vi "CtlRefToJson.vi"(8 "error (in)":errorcluster, 10 "Destination Directory":path, 11 "vi reference":refnum<vi>) -> (0 "error out":errorcluster, 1 "JSON File Path":path, 3 "String":string)   [LabVIEW 2017]
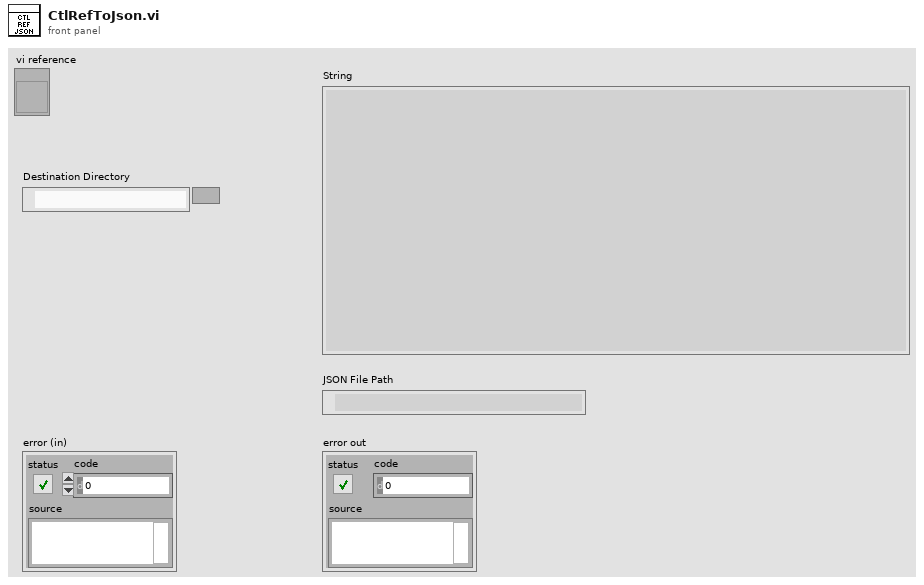
[diagram p1: front panel]
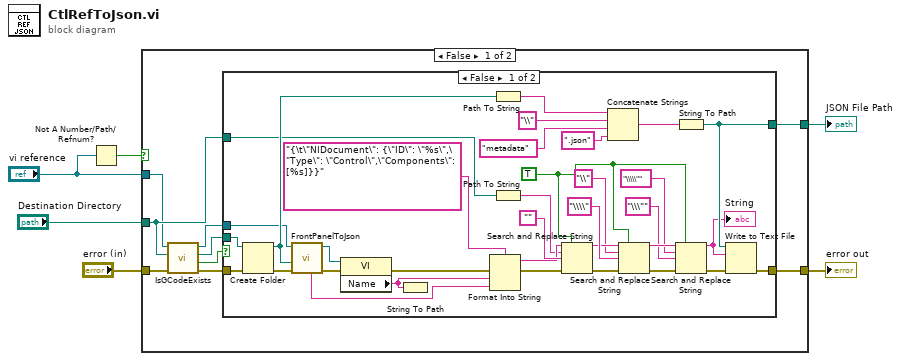
[diagram p0: block diagram]
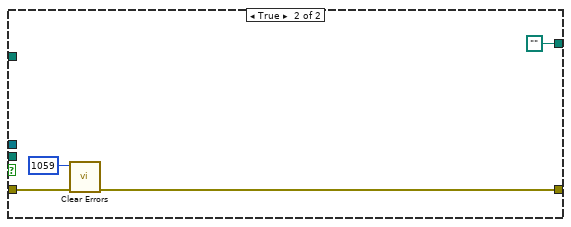
[diagram p2: hidden frame]
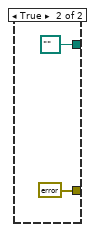
[diagram p3: hidden frame]
diagram:
  n1 = Not A Number/Path/Refnum?(number/path/refnum="vi reference") -> (NaN/Path/Refnum?=w2:bool)
  n2 = case shown="False" w2 {
    tunnel: [w15 path ""] -> w6
    tunnel: [w14 errorcluster {"status"=FALSE, "code"=0, "source"=""} ("error out")] -> w5
    tunnel: "error (in)" -> [w13 _]
    tunnel: "Destination Directory" -> [w10 _]
    tunnel: "vi reference" -> [w9 _]
    frame False {
      n3 = call "IsGCodeExists.vi"("error in (no error)"=w13, "Destination Directory"=w10, "VI (in)"=w9) -> ("error out"=w11:errorcluster, "file or folder exists?"=w12:bool, "VI Folder"=w7:path, "VI (out)"=w8:refnum<vi>)  [unwired: 3 in]
      n4 = case shown="False" w12 {
        tunnel: [w49 path ""] -> w15
        tunnel: [w27 w53] -> w14
        tunnel: w10 -> [w20 _]
        tunnel: w8 -> [w30 _]
        tunnel: w11 -> [w29 w50]
        tunnel: w7 -> [w28 _]
        frame False {
          w21 = TRUE ("replace all? (F)")
          n5 = Create Folder(path (use dialog)=w28, error in=w29) -> (created path=w34:path, error out=w32:errorcluster)  [unwired: 1 in, 1 out]
          n6 = call "FrontPanelToJson.vi"("error in"=w32, "VI Path"=w34, "VI in"=w30) -> ("error out"=w31:errorcluster, "VI out"=w18:refnum<vi>, "JSON"=w33:string)  [unwired: 5 in]
          n7 = property class="VI"(reference=w18, error in=w31) -> (error out=w40:errorcluster, "Name"=w17:string)  [unwired: 1 out]
          n8 = String To Path(string=w17) -> ()  [unwired: 1 out]
          n9 = Format Into String(format string="{\t\"NIDocument\": {\"ID\": \"%s\",\"Type\": \"Control\",\"Components\": [%s]}}", error in=w40, w17, w33) -> (resulting string=w44:string, error out=w38:errorcluster)  [unwired: 1 in]
          n10 = Path To String(path=w34) -> (string=w39:string)
          n11 = Path To String(path=w20) -> (string=w35:string)
          n12 = Search and Replace String(replace all?=w21, input string=w44, search string=w35, replace string="", error in=w38) -> (result string=w45:string, error out=w37:errorcluster)  [unwired: 3 in, 2 out]
          n13 = Concatenate Strings(w39, "\\" ("string"), "metadata" ("string"), ".json" ("string")) -> (w48:string)
          n14 = Search and Replace String(replace all?=w21, input string=w45, search string="\\", replace string="\\\\" ("replace string (\"\")"), error in=w37) -> (result string=w26:string, error out=w22:errorcluster)  [unwired: 3 in, 2 out]
          n15 = String To Path(string=w48) -> (path=w49:path)
          n16 = Search and Replace String(replace all?=w21, input string=w26, search string="\\\\\"", replace string="\\\"" ("replace string (\"\")"), error in=w22) -> (result string=w25:string, error out=w19:errorcluster)  [unwired: 3 in, 2 out]
          "String" <- w25
          n17 = Write to Text File(file (use dialog)=w49, text=w25, error in=w19) -> (error out=w27:errorcluster)  [unwired: 1 in, 2 out]
        }
        frame True {
          n18 = call <vilib>:"Clear Errors.vi"("error in (no error)"=w50, "specific error code to clear (0: all)"=1059) -> ("error out"=w53:errorcluster)  [unwired: 4 in, 1 out]
        }
      }
    }
    frame True {
    }
  }
  "JSON File Path" <- w6
  "error out" <- w5
